vi "oa_Check Vector Reference is Empty (N Channels).vi"(0 "magnitudes [RMS] in":T1(array[cluster]) {"magnitude" format="%.2f"; "time/rev/rpm" format="%.2f"}, 2 "reset? (F)":bool, 5 "phases [phase lag] in":cluster{"time/rev/rpm":dbl[], "phase":dbl[]}[][](array[cluster]) {"phase" format="%.2f"; "time/rev/rpm" format="%.2f"}, 11 "error in (no error)":errorcluster) -> (4 "magnitudes [RMS] out":T1(array[cluster]) {"magnitude" format="%.2f"; "time/rev/rpm" format="%.2f"}, 6 "phases [phase lag] out":cluster{"time/rev/rpm":dbl[], "phase":dbl[]}[][](array[cluster]) {"phase" format="%.2f"; "time/rev/rpm" format="%.2f"}, 8 "empty?":bool, 15 "error out":errorcluster)   [LabVIEW 2017, in "SoundVib_RefDataProcess.lvlib"]
uses:
  <vilib>/addons/Sound and Vibration/Order Analysis/Referece Data Processing/SoundVib_RefDataProcess.lvlib
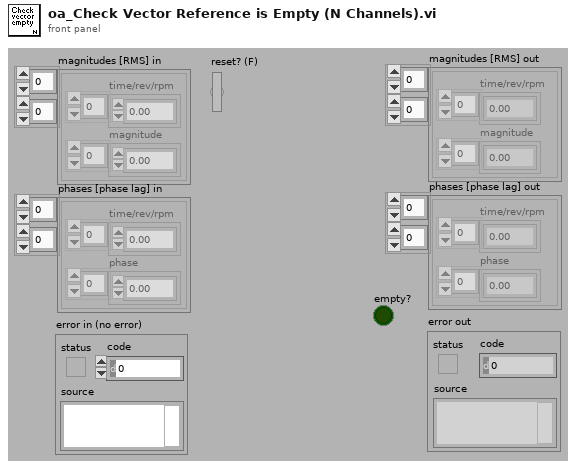
[diagram p1: front panel]
types:
  T1 = cluster{"time/rev/rpm":dbl[], "magnitude":dbl[]}[][]
  T2 = cluster{"is warning? (False)":bool, "error code (0)":i32, "error message (\"\")":string}
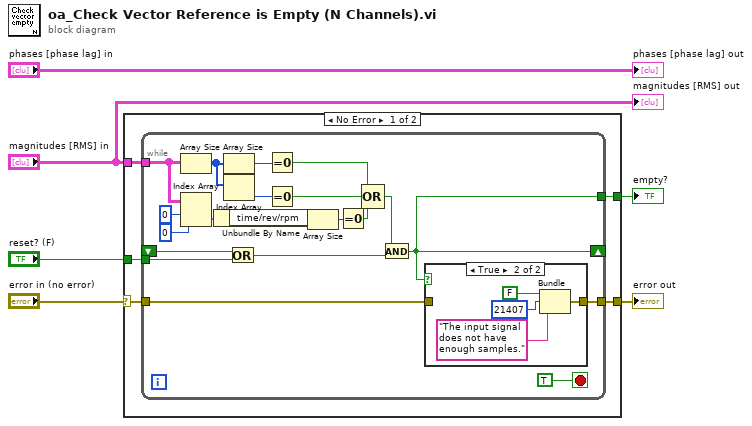
[diagram p0: block diagram]
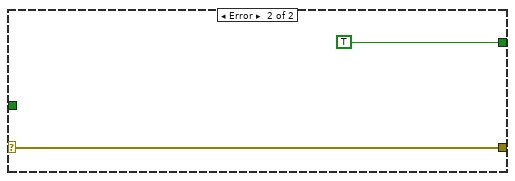
[diagram p3: hidden frame]
diagram:
  n1 = case shown="No Error" "error in (no error)" {
    selector: "error in (no error)" -> [w10 w37]
    tunnel: "magnitudes [RMS] in" -> [w11 _]
    tunnel: [w8 TRUE] -> w4
    tunnel: [w9 w37] -> w2
    tunnel: "reset? (F)" -> [w7 _]
    frame No Error {
      n2 = while {
        tunnel: w11 -> [w31]
        tunnel: w10 -> [w26]
        tunnel: [w25] -> w9
        tunnel: [w12] -> w8
        shift-right: [w12] -> _
        shift-left: _ -> [w15]
        tunnel: w7 -> [w16]
        stop <- TRUE stop-if-true
        n3 = Array Size(array=w31) -> (size(s)=w20:i32[])
        n4 = Index Array(array=w31, index (row)=0, index (col)=0 ("disabled index (col)")) -> (element=w30:cluster{"time/rev/rpm":dbl[], "magnitude":dbl[]})
        n5 = Unbundle By Name(w30) -> ("time/rev/rpm"=w29:dbl[])
        n6 = Array Size(array=w20) -> (size(s)=w19:i32)
        n7 = Index Array(array=w20) -> (element=w22:i32)  [unwired: 1 in]
        n8 = Or(x=w15, y=w16) -> (x .or. y?=w14:bool)
        n9 = Equal To 0?(x=w19) -> (x = 0?=w18:bool)
        n10 = Equal To 0?(x=w22) -> (x = 0?=w21:bool)
        n11 = Array Size(array=w29) -> (size(s)=w27:i32)
        n12 = Equal To 0?(x=w27) -> (x = 0?=w28:bool)
        n13 = Compound Arithmetic op=OR(w18, w21, w28) -> (w13:bool)
        n14 = And(x=w13, y=w14) -> (x .and. y?=w12:bool)
        n15 = case shown="True" w12 {
          tunnel: w26 -> [w32 _]
          tunnel: [w32 w33] -> w25
          frame False {
          }
          frame True {
            n16 = Bundle("is warning? (False)"=FALSE, "error code (0)"=21407, "error message (\"\")"="The input signal does not have enough samples." ("error message (\"\")")) -> (w33:T2)  [unwired: 1 in]
          }
        }
      }
    }
    frame Error {
    }
  }
  "empty?" <- w4
  "error out" <- w2
  "magnitudes [RMS] out" <- "magnitudes [RMS] in"
  "phases [phase lag] out" <- "phases [phase lag] in"
